vi "GV PockelsMainDelay_tick.vi"() -> ()   [LabVIEW 2017]
panel:
  out "PockelsFirstFrameDelay_tick":u32
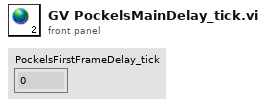
[diagram p1: front panel]
diagram:
